vi "UI_Unlock_(02).vi"(3 "error in (no error)":errorcluster, 4 "Settings cluster in":T1={"Defaults"={"Default User"=0.0, "VISA Resource Name "=""}, "Recording and saving"={"Researcher name"="", "Name prefix"="", "Data filtering"=0, "Stop at"=0.0, "\"Stop at\" enabled"=FALSE}, "Geometry"={"Cage diameter, mm"=0, "Starting angle MIDFIELD"=0, "Starting angle BORDER"=0, "Radius, mm CENTER"=0, "Radius, mm MIDFIELD"=0, "N segments MIDFIELD"=0, "N segments BORDER"=0, "R-gap, mm"=0.0, "Bridge swap"=FALSE, "Bridge H. offset"=0.0, "Bridge V. offset"=0.0, "Twisted neck"=FALSE}, "IO parameters"={"IO general config."=0, "IO 1 configuration"=0, "IO 2 configuration"=0, "IO 3 configuration"=0, "IO 4 configuration"=0, "Activate ext. RS-232"=0, "IO inversion config."=0, "Sync capability"=1}, "Stimulus presets array"=[{"Event type"=0, "Dur., s"=0.0, "Stim., s"=0.0, "TTL out N"=1, "Set/Clear"=FALSE, "Stim. has been set"=FALSE}, {"Event type"=0, "Dur., s"=0.0, "Stim., s"=0.0, "TTL out N"=1, "Set/Clear"=FALSE, "Stim. has been set"=FALSE}, {"Event type"=0, "Dur., s"=0.0, "Stim., s"=0.0, "TTL out N"=1, "Set/Clear"=FALSE, "Stim. has been set"=FALSE}, {"Event type"=0, "Dur., s"=0.0, "Stim., s"=0.0, "TTL out N"=1, "Set/Clear"=FALSE, "Stim. has been set"=FALSE}, {"Event type"=0, "Dur., s"=0.0, "Stim., s"=0.0, "TTL out N"=1, "Set/Clear"=FALSE, "Stim. has been set"=FALSE}, {"Event type"=0, "Dur., s"=0.0, "Stim., s"=0.0, "TTL out N"=1, "Set/Clear"=FALSE, "Stim. has been set"=FALSE}, {"Event type"=0, "Dur., s"=0.0, "Stim., s"=0.0, "TTL out N"=1, "Set/Clear"=FALSE, "Stim. has been set"=FALSE}, {"Event type"=0, "Dur., s"=0.0, "Stim., s"=0.0, "TTL out N"=1, "Set/Clear"=FALSE, "Stim. has been set"=FALSE}, {"Event type"=0, "Dur., s"=0.0, "Stim., s"=0.0, "TTL out N"=1, "Set/Clear"=FALSE, "Stim. has been set"=FALSE}, {"Event type"=0, "Dur., s"=0.0, "Stim., s"=0.0, "TTL out N"=1, "Set/Clear"=FALSE, "Stim. has been set"=FALSE}, {"Event type"=0, "Dur., s"=0.0, "Stim., s"=0.0, "TTL out N"=1, "Set/Clear"=FALSE, "Stim. has been set"=FALSE}, {"Event type"=0, "Dur., s"=0.0, "Stim., s"=0.0, "TTL out N"=1, "Set/Clear"=FALSE, "Stim. has been set"=FALSE}, {"Event type"=0, "Dur., s"=0.0, "Stim., s"=0.0, "TTL out N"=1, "Set/Clear"=FALSE, "Stim. has been set"=FALSE}, {"Event type"=0, "Dur., s"=0.0, "Stim., s"=0.0, "TTL out N"=1, "Set/Clear"=FALSE, "Stim. has been set"=FALSE}], "Settings loaded OK"=FALSE} {"Stimulus presets array"."Event type" items=["Stay for N seconds"]; "Stimulus presets array"."TTL out N" items=["1"=1, "2"=2, "1+2"=3]; "Geometry"."Cage diameter, mm" scale=0.0..340.0}, 5 "All references in":T6) -> (0 "error out":errorcluster, 1 "Settings cluster out":T1={"Defaults"={"Default User"=0.0, "VISA Resource Name "=""}, "Recording and saving"={"Researcher name"="", "Name prefix"="", "Data filtering"=0, "Stop at"=0.0, "\"Stop at\" enabled"=FALSE}, "Geometry"={"Cage diameter, mm"=0, "Starting angle MIDFIELD"=0, "Starting angle BORDER"=0, "Radius, mm CENTER"=0, "Radius, mm MIDFIELD"=0, "N segments MIDFIELD"=0, "N segments BORDER"=0, "R-gap, mm"=0.0, "Bridge swap"=FALSE, "Bridge H. offset"=0.0, "Bridge V. offset"=0.0, "Twisted neck"=FALSE}, "IO parameters"={"IO general config."=0, "IO 1 configuration"=0, "IO 2 configuration"=0, "IO 3 configuration"=0, "IO 4 configuration"=0, "Activate ext. RS-232"=0, "IO inversion config."=0, "Sync capability"=1}, "Stimulus presets array"=[{"Event type"=0, "Dur., s"=0.0, "Stim., s"=0.0, "TTL out N"=1, "Set/Clear"=FALSE, "Stim. has been set"=FALSE}, {"Event type"=0, "Dur., s"=0.0, "Stim., s"=0.0, "TTL out N"=1, "Set/Clear"=FALSE, "Stim. has been set"=FALSE}, {"Event type"=0, "Dur., s"=0.0, "Stim., s"=0.0, "TTL out N"=1, "Set/Clear"=FALSE, "Stim. has been set"=FALSE}, {"Event type"=0, "Dur., s"=0.0, "Stim., s"=0.0, "TTL out N"=1, "Set/Clear"=FALSE, "Stim. has been set"=FALSE}, {"Event type"=0, "Dur., s"=0.0, "Stim., s"=0.0, "TTL out N"=1, "Set/Clear"=FALSE, "Stim. has been set"=FALSE}, {"Event type"=0, "Dur., s"=0.0, "Stim., s"=0.0, "TTL out N"=1, "Set/Clear"=FALSE, "Stim. has been set"=FALSE}, {"Event type"=0, "Dur., s"=0.0, "Stim., s"=0.0, "TTL out N"=1, "Set/Clear"=FALSE, "Stim. has been set"=FALSE}, {"Event type"=0, "Dur., s"=0.0, "Stim., s"=0.0, "TTL out N"=1, "Set/Clear"=FALSE, "Stim. has been set"=FALSE}, {"Event type"=0, "Dur., s"=0.0, "Stim., s"=0.0, "TTL out N"=1, "Set/Clear"=FALSE, "Stim. has been set"=FALSE}, {"Event type"=0, "Dur., s"=0.0, "Stim., s"=0.0, "TTL out N"=1, "Set/Clear"=FALSE, "Stim. has been set"=FALSE}, {"Event type"=0, "Dur., s"=0.0, "Stim., s"=0.0, "TTL out N"=1, "Set/Clear"=FALSE, "Stim. has been set"=FALSE}, {"Event type"=0, "Dur., s"=0.0, "Stim., s"=0.0, "TTL out N"=1, "Set/Clear"=FALSE, "Stim. has been set"=FALSE}, {"Event type"=0, "Dur., s"=0.0, "Stim., s"=0.0, "TTL out N"=1, "Set/Clear"=FALSE, "Stim. has been set"=FALSE}, {"Event type"=0, "Dur., s"=0.0, "Stim., s"=0.0, "TTL out N"=1, "Set/Clear"=FALSE, "Stim. has been set"=FALSE}], "Settings loaded OK"=FALSE} {"Stimulus presets array"."Event type" items=["Stay for N seconds"]; "Stimulus presets array"."TTL out N" items=["1"=1, "2"=2, "1+2"=3]; "Geometry"."Cage diameter, mm" scale=0.0..340.0}, 2 "All references out":T6)   [LabVIEW 2018]
uses:
  Controls/CTL_All_References.ctl
  Controls/CTL_Controls_References.ctl
  Controls/CTL_Indicators_References.ctl
  Controls/CTL_Panes_and_VIs_References.ctl
  Controls/CTL_Histogram_Properties.ctl
  <vilib>/Utility/miscctls.llb/LVRangeTypeDef.ctl
  Controls/CTL_Settings_cluster.ctl
  Controls/CTL_IO_params_cluster.ctl
  Controls/CTL_Single_stimulus_setting.ctl
  <vilib>/Utility/error.llb/Error Cluster From Error Code.vi
  <vilib>/ErrorRing/Error Ring.xnode
panel:
  in  "Histogram initialization cluster":T4={"X Scale.Range"={"Minimum"=0.0, "Maximum"=13.0, "Increment"=1.0, "Minor Increment"=1.0, "Start"=0.0}, "Caption.Text"="Zone preference (normalized)", "X Scale.Offset and Multiplier:Multiplier"=1.0, "X Scale.Offset and Multiplier:Offset"=0.0, "X Scale.Scale Fit"=2, "X Scale.Display Format:Precision"=0, "Y Scale.Mapping Mode"=0, "Zones preference empty initialized array"=[0, 0, 0, 0, 0, 0, 0, 0, 0, 0, 0, 0, 0, 0], "Plot.Fill/Point Color"=15790320}
  out "Panes references":T9
  out "Controls references params":string[][](array[string])
  out "Indicators references params":string[][](array[string])
  out "Indicators references":T8
  out "Controls references":T7
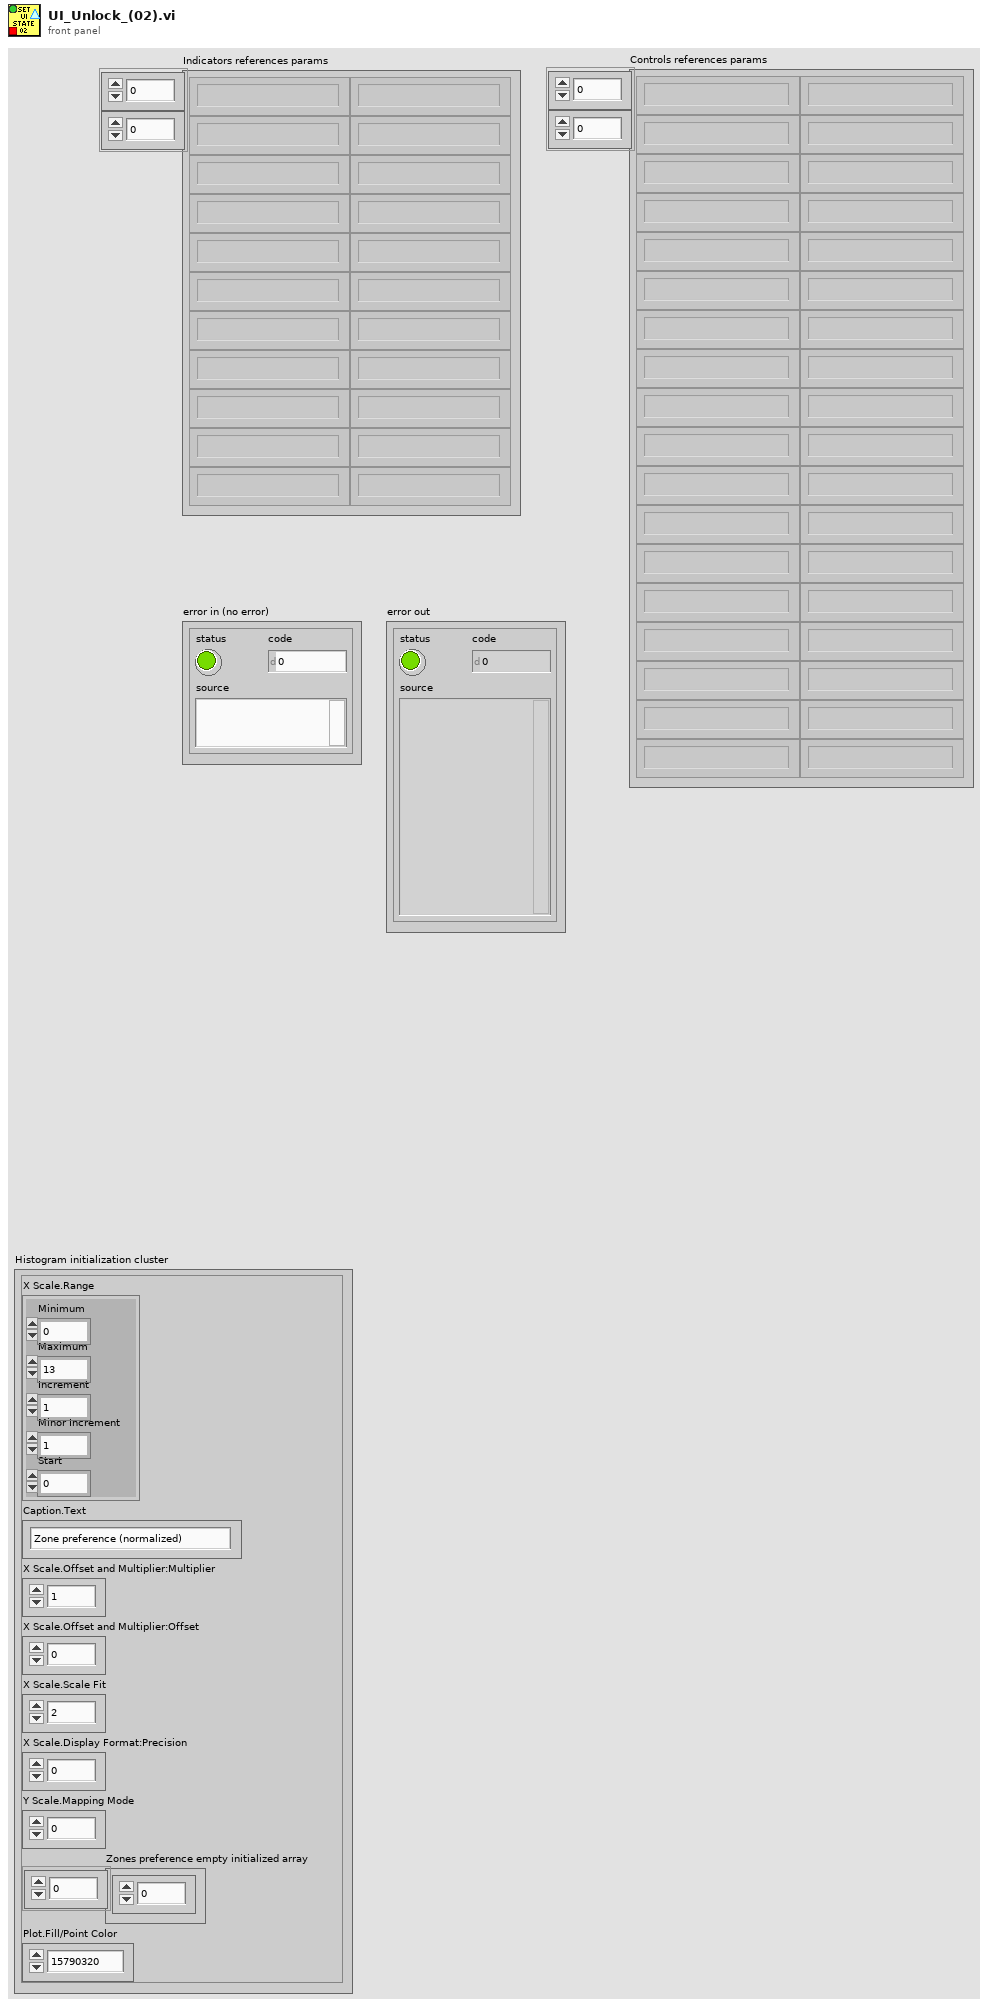
[diagram p1: front panel]
types:
  T1 = typedef "CTL_Settings_cluster.ctl" = cluster{"Defaults":cluster{"Default User":dbl, "VISA Resource Name ":string}, "Recording and saving":cluster{"Researcher name":string, "Name prefix":string, "Data filtering":u16, "Stop at":dbl, "\"Stop at\" enabled":bool}, "Geometry":cluster{"Cage diameter, mm":u16, "Starting angle MIDFIELD":i16, "Starting angle BORDER":i16, "Radius, mm CENTER":u16, "Radius, mm MIDFIELD":u16, "N segments MIDFIELD":u8, "N segments BORDER":u8, "R-gap, mm":sgl, "Bridge swap":bool, "Bridge H. offset":sgl, "Bridge V. offset":sgl, "Twisted neck":bool}, "IO parameters":T2, "Stimulus presets array":T3[], "Settings loaded OK":bool}
  T2 = typedef "CTL_IO_params_cluster.ctl" = cluster{"IO general config.":u16, "IO 1 configuration":u16, "IO 2 configuration":u16, "IO 3 configuration":u16, "IO 4 configuration":u16, "Activate ext. RS-232":u16, "IO inversion config.":u16, "Sync capability":u8}
  T3 = typedef "CTL_Single_stimulus_setting.ctl" = cluster{"Event type":u16, "Dur., s":sgl, "Stim., s":sgl, "TTL out N":u16, "Set/Clear":bool, "Stim. has been set":bool}
  T4 = typedef "CTL_Histogram_Properties.ctl" = cluster{"X Scale.Range":T5, "Caption.Text":string, "X Scale.Offset and Multiplier:Multiplier":dbl, "X Scale.Offset and Multiplier:Offset":dbl, "X Scale.Scale Fit":u8, "X Scale.Display Format:Precision":u8, "Y Scale.Mapping Mode":u8, "Zones preference empty initialized array":i32[], "Plot.Fill/Point Color":u32}
  T5 = typedef "LVRangeTypeDef.ctl" = cluster{"Minimum":dbl, "Maximum":dbl, "Increment":dbl, "Minor Increment":dbl, "Start":dbl}
  T6 = typedef "CTL_All_References.ctl" = cluster{"Controls references":T7, "Indicators references":T8, "Panes references":T9}
  T7 = typedef "CTL_Controls_References.ctl" = cluster{"Check HW connection":refnum<vi>, "Start Tracking button":refnum<vi>, "Reset zones":refnum<vi>, "Reset stimuli":refnum<vi>, "Record/Stop":refnum<vi>, "Reset barplot":refnum<vi>, "Multiplyer of chart RX":refnum<vi>, "Show zones":refnum<vi>, "Show magnets":refnum<vi>, "Show heatmap":refnum<vi>, "Show full track":refnum<vi>, "Open File":refnum<vi>, "Play/Pause":refnum<vi>, "Trace, s":refnum<vi>, "Playback speed":refnum<vi>, "Timeline":refnum<vi>, "By Zone stim. setup":refnum<vi>, "Set, Rec and Analyse Tab":refnum<vi>, "Cage radial segmentation":refnum<vi>, "Set IO config":refnum<vi>}
  T8 = typedef "CTL_Indicators_References.ctl" = cluster{"HW info":refnum<vi>, "Port":refnum<vi>, "Ready":refnum<vi>, "IO status indicator":refnum<vi>, "Current Time":refnum<vi>, "Record timestamp":refnum<vi>, "Mouse speed":refnum<vi>, "Mouse speed, mm/s":refnum<vi>, "Running, perc. of time":refnum<vi>, "Histograms":refnum<vi>}
  T9 = typedef "CTL_Panes_and_VIs_References.ctl" = cluster{"Pane":refnum<vi>, "This VI":refnum<vi>}
  T10 = cluster{"Cage diameter, mm":u16, "Starting angle MIDFIELD":i16, "Starting angle BORDER":i16, "Radius, mm CENTER":u16, "Radius, mm MIDFIELD":u16, "N segments MIDFIELD":u8, "N segments BORDER":u8, "R-gap, mm":sgl, "Bridge swap":bool, "Bridge H. offset":sgl, "Bridge V. offset":sgl, "Twisted neck":bool}
  T11 = enum8{"Enabled", "Disabled", "Disabled and Grayed Out"}
  T12 = enum32{"Page Enabled", "Page Disabled", "Page Disabled & Grayed"}
  T13 = cluster{"Radius, mm MIDFIELD":u16, "N segments MIDFIELD":u8, "Starting angle MIDFIELD":i16}
  T14 = cluster{"N segments BORDER":u8, "Starting angle BORDER":i16}
  T15 = cluster{cluster{"Radius, mm CENTER":u16}, cluster{"Radius, mm MIDFIELD":u16, "N segments MIDFIELD":u8, "Starting angle MIDFIELD":i16}, cluster{"N segments BORDER":u8, "Starting angle BORDER":i16}}
  T16 = typedef "CTL_IO_parameters_indicator.ctl" = cluster{"IO1":bool, "IO2":bool, "IO3":bool, "IO4":bool, "Z1":bool, "Z2":bool, "Z3":bool, "Z4":bool, "St1":bool, "St2":bool, "St3":bool, "St4":bool, "Syn1":bool, "Syn2":bool, "RS-232 ext. activated":bool}
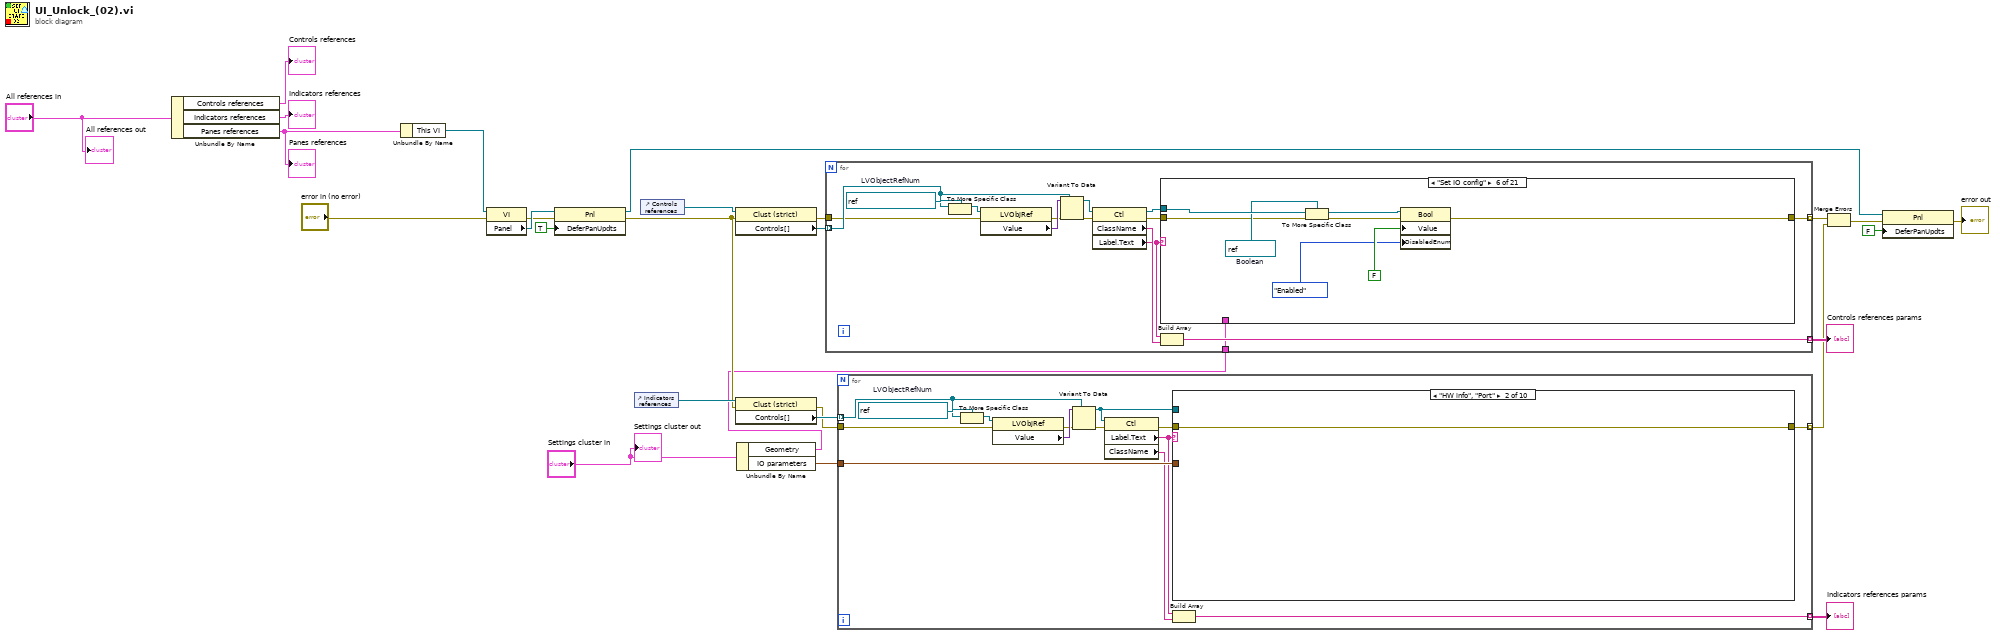
[diagram p0: block diagram]
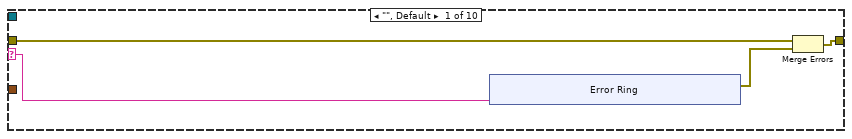
[diagram p2: hidden frame]
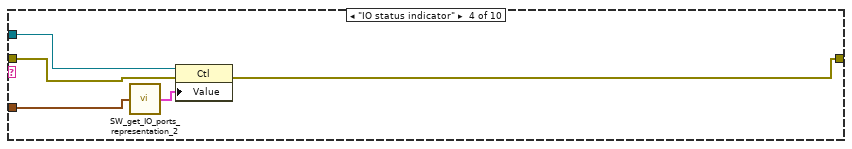
[diagram p4: hidden frame]
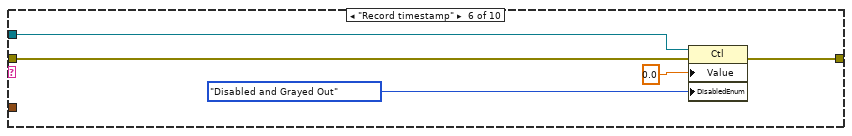
[diagram p6: hidden frame]
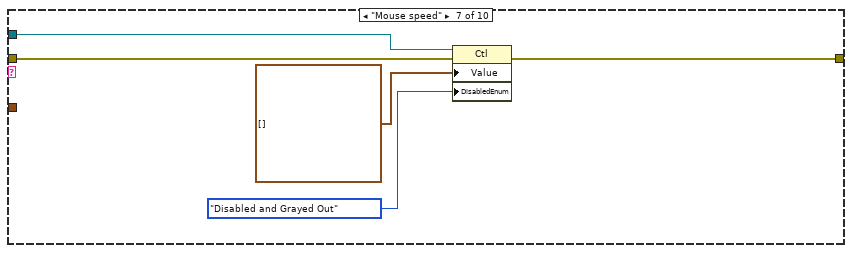
[diagram p7: hidden frame]
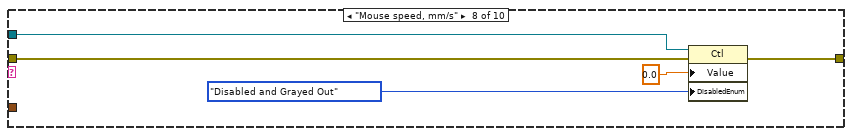
[diagram p8: hidden frame]
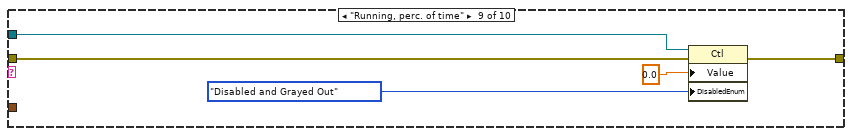
[diagram p9: hidden frame]
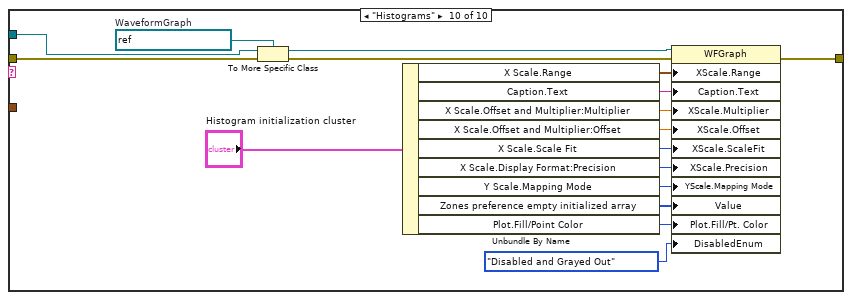
[diagram p10: hidden frame]
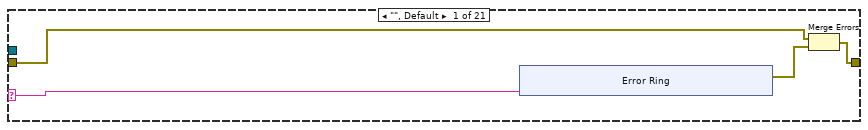
[diagram p11: hidden frame]
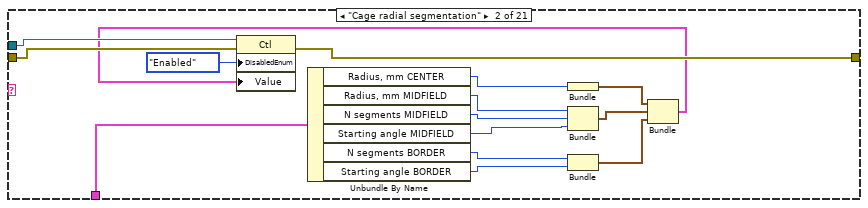
[diagram p12: hidden frame]
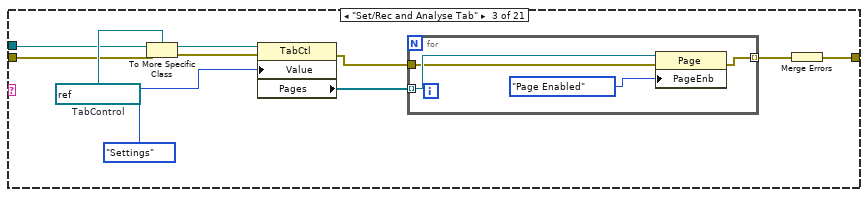
[diagram p13: hidden frame]
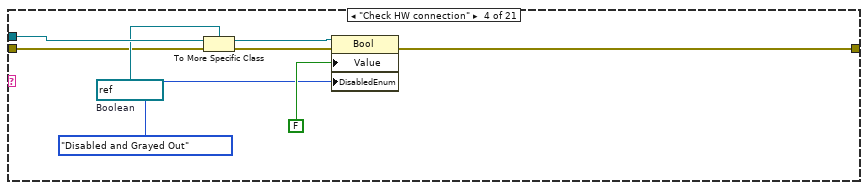
[diagram p14: hidden frame]
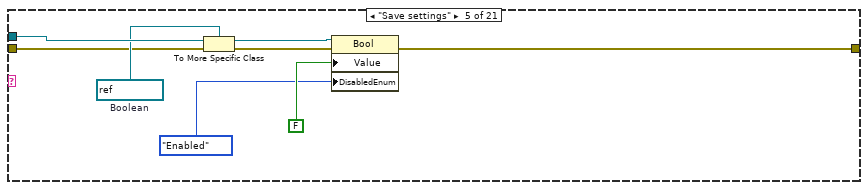
[diagram p15: hidden frame]
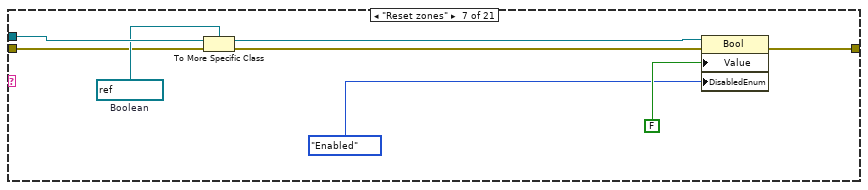
[diagram p16: hidden frame]
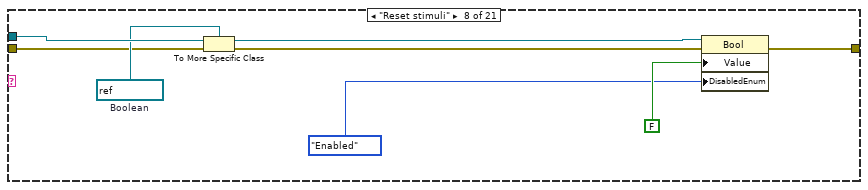
[diagram p17: hidden frame]
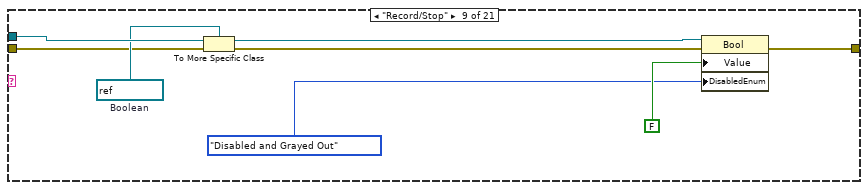
[diagram p18: hidden frame]
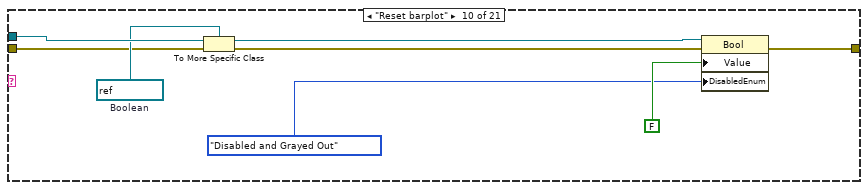
[diagram p19: hidden frame]
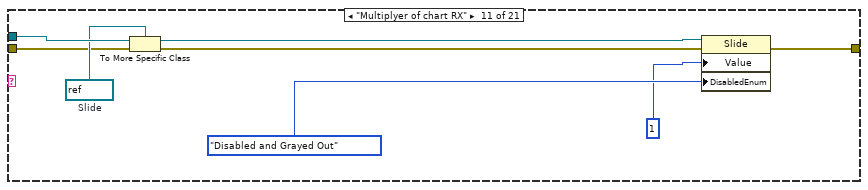
[diagram p20: hidden frame]
diagram:
  n1 = Unbundle By Name("All references in") -> ("Controls references"=→"Controls references":T7, "Indicators references"=→"Indicators references":T8, "Panes references"=w18:T9)
  "Panes references" <- w18
  n2 = Unbundle By Name(w18) -> ("This VI"=w15:refnum<vi>)
  n3 = property class="VI"(reference=w15, error in="error in (no error)") -> (error out=w7:errorcluster, "Panel"=w17:refnum<vi>)  [unwired: 1 out]
  n4 = property class="Pnl"(reference=w17, error in=w7, "DeferPanUpdts"=TRUE ("Defer Panel Updates")) -> (reference out=w8:refnum<vi>, error out=w14:errorcluster)
  n5 = control-ref of="Indicators references"() -> (w21:refnum<vi>)
  n6 = control-ref of="Controls references"() -> (w23:refnum<vi>)
  n7 = property class="Clust (strict)"(reference=w23, error in=w14) -> (error out=w13:errorcluster, "Controls[]"=w24:refnum<vi>[])  [unwired: 1 out]
  n8 = property class="Clust (strict)"(reference=w21, error in=w14) -> (error out=w12:errorcluster, "Controls[]"=w22:refnum<vi>[])  [unwired: 1 out]
  n9 = Unbundle By Name("Settings cluster in") -> ("Geometry"=w1:T10, "IO parameters"=w3:T2)
  n10 = for {
    tunnel: w24 -> [w39] mode=indexing
    tunnel: [w36] -> w19 mode=indexing
    tunnel: w13 -> [w35]
    tunnel: [w31] -> w5 mode=indexing
    tunnel: w1 -> [w28]
    w41 = refnum<vi> refnum  # LVObjectRefNum
    n11 = To More Specific Class(target class=w41, reference=w39) -> (specific class reference=w42:refnum<vi>)  [unwired: 1 in, 1 out]
    n12 = property class="LVObjRef"(reference=w42, error in=w35) -> (error out=w34:errorcluster, "Value"=w40:variant)  [unwired: 1 out]
    n13 = Variant To Data(error in=w34, type=w39, Variant=w40) -> (data=w38:refnum<vi>, error out=w33:errorcluster)
    n14 = property class="Ctl"(reference=w38, error in=w33) -> (reference out=w29:refnum<vi>, error out=w30:errorcluster, "ClassName"=w37:string, "Label.Text"=w32:string)
    n15 = case shown="\"Set IO config\"" w32 {
      selector: w32 -> [w43 _ _ _ _ _ _ _ _ _ _ _ _ _ _ _ _ _ _ _ _]
      tunnel: [w45 w66 w69 w85 w93 w101 w109 w117 w125 w133 w141 w149 w157 w165 w173 w181 w189 w197 w205 w213 w220] -> w31
      tunnel: w30 -> [w46 w67 w70 w87 w95 w103 w111 w119 w127 w135 w143 w151 w159 w167 w175 w183 w191 w199 w207 w215 w222]
      tunnel: w29 -> [_ w68 w71 w90 w98 w106 w114 w122 w130 w138 w146 w154 w162 w170 w178 w186 w194 w202 w210 w218 w225]
      tunnel: w28 -> [_ w64 _ _ _ _ _ _ _ _ _ _ _ _ _ _ _ _ _ _ _]
      frame "", Default {
        n16 = xnode "Error Ring"("parameter 0"=w43) -> ("error out"=w44:errorcluster)
        n17 = Merge Errors(w46, w44) -> (w45:errorcluster)
      }
      frame "Cage radial segmentation" {
        n18 = Unbundle By Name(w64) -> ("Radius, mm CENTER"=w63:u16, "Radius, mm MIDFIELD"=w62:u16, "N segments MIDFIELD"=w61:u8, "Starting angle MIDFIELD"=w60:i16, "N segments BORDER"=w59:u8, "Starting angle BORDER"=w58:i16)
        n19 = Bundle("Radius, mm CENTER"=w63) -> (w57:cluster{"Radius, mm CENTER":u16})  [unwired: 1 in]
        n20 = Bundle("Radius, mm MIDFIELD"=w62, "N segments MIDFIELD"=w61, "Starting angle MIDFIELD"=w60) -> (w56:T13)  [unwired: 1 in]
        n21 = Bundle("N segments BORDER"=w59, "Starting angle BORDER"=w58) -> (w55:T14)  [unwired: 1 in]
        n22 = Bundle(w57, w56, w55) -> (w54:T15)  [unwired: 1 in]
        n23 = property class="Ctl"(reference=w68, error in=w67, "DisabledEnum"=T11."Enabled" ("Disabled"), "Value"=w54) -> (error out=w66:errorcluster)  [unwired: 1 out]
      }
      frame "Set/Rec and Analyse Tab" {
        w76 = refnum<vi> refnum  # TabControl
        n24 = To More Specific Class(target class=w76, reference=w71, error in=w70) -> (specific class reference=w77:refnum<vi>, error out=w74:errorcluster)
        n25 = property class="TabCtl"(reference=w77, error in=w74, "Value"=enum32{"Settings", "Recording and Analysis"}."Settings") -> (error out=w73:errorcluster, "Pages"=w75:refnum<vi>[])  [unwired: 1 out]
        n26 = for {
          tunnel: w75 -> [w81] mode=indexing
          tunnel: w73 -> [w80]
          tunnel: [w79] -> w72 mode=indexing
          n27 = property class="Page"(reference=w81, error in=w80, "PageEnb"=T12."Page Enabled" ("Page Enabled State")) -> (error out=w79:errorcluster)  [unwired: 1 out]
        }
        n28 = Merge Errors(w72) -> (w69:errorcluster)
      }
      frame "Check HW connection" {
        w89 = refnum<vi> refnum  # Boolean
        n29 = To More Specific Class(target class=w89, reference=w90, error in=w87) -> (specific class reference=w88:refnum<vi>, error out=w86:errorcluster)
        n30 = property class="Bool"(reference=w88, error in=w86, "Value"=FALSE, "DisabledEnum"=T11."Disabled and Grayed Out" ("Disabled")) -> (error out=w85:errorcluster)  [unwired: 1 out]
      }
      frame "Save settings" {
        w97 = refnum<vi> refnum  # Boolean
        n31 = To More Specific Class(target class=w97, reference=w98, error in=w95) -> (specific class reference=w96:refnum<vi>, error out=w94:errorcluster)
        n32 = property class="Bool"(reference=w96, error in=w94, "Value"=FALSE, "DisabledEnum"=T11."Enabled" ("Disabled")) -> (error out=w93:errorcluster)  [unwired: 1 out]
      }
      frame "Set IO config" {
        w105 = refnum<vi> refnum  # Boolean
        n33 = To More Specific Class(target class=w105, reference=w106, error in=w103) -> (specific class reference=w104:refnum<vi>, error out=w102:errorcluster)
        n34 = property class="Bool"(reference=w104, error in=w102, "Value"=FALSE, "DisabledEnum"=T11."Enabled" ("Disabled")) -> (error out=w101:errorcluster)  [unwired: 1 out]
      }
      frame "Reset zones" {
        w113 = refnum<vi> refnum  # Boolean
        n35 = To More Specific Class(target class=w113, reference=w114, error in=w111) -> (specific class reference=w112:refnum<vi>, error out=w110:errorcluster)
        n36 = property class="Bool"(reference=w112, error in=w110, "Value"=FALSE, "DisabledEnum"=T11."Enabled" ("Disabled")) -> (error out=w109:errorcluster)  [unwired: 1 out]
      }
      frame "Reset stimuli" {
        w121 = refnum<vi> refnum  # Boolean
        n37 = To More Specific Class(target class=w121, reference=w122, error in=w119) -> (specific class reference=w120:refnum<vi>, error out=w118:errorcluster)
        n38 = property class="Bool"(reference=w120, error in=w118, "Value"=FALSE, "DisabledEnum"=T11."Enabled" ("Disabled")) -> (error out=w117:errorcluster)  [unwired: 1 out]
      }
      frame "Record/Stop" {
        w129 = refnum<vi> refnum  # Boolean
        n39 = To More Specific Class(target class=w129, reference=w130, error in=w127) -> (specific class reference=w128:refnum<vi>, error out=w126:errorcluster)
        n40 = property class="Bool"(reference=w128, error in=w126, "Value"=FALSE, "DisabledEnum"=T11."Disabled and Grayed Out" ("Disabled")) -> (error out=w125:errorcluster)  [unwired: 1 out]
      }
      frame "Reset barplot" {
        w137 = refnum<vi> refnum  # Boolean
        n41 = To More Specific Class(target class=w137, reference=w138, error in=w135) -> (specific class reference=w136:refnum<vi>, error out=w134:errorcluster)
        n42 = property class="Bool"(reference=w136, error in=w134, "Value"=FALSE, "DisabledEnum"=T11."Disabled and Grayed Out" ("Disabled")) -> (error out=w133:errorcluster)  [unwired: 1 out]
      }
      frame "Multiplyer of chart RX" {
        w145 = refnum<vi> refnum  # Slide
        n43 = To More Specific Class(target class=w145, reference=w146, error in=w143) -> (specific class reference=w144:refnum<vi>, error out=w142:errorcluster)
        n44 = property class="Slide"(reference=w144, error in=w142, "Value"=u8 1, "DisabledEnum"=T11."Disabled and Grayed Out" ("Disabled")) -> (error out=w141:errorcluster)  [unwired: 1 out]
      }
      frame "Show zones" {
        w153 = refnum<vi> refnum  # Boolean
        n45 = To More Specific Class(target class=w153, reference=w154, error in=w151) -> (specific class reference=w152:refnum<vi>, error out=w150:errorcluster)
        n46 = property class="Bool"(reference=w152, error in=w150, "Value"=TRUE, "DisabledEnum"=T11."Enabled" ("Disabled")) -> (error out=w149:errorcluster)  [unwired: 1 out]
      }
      frame "Show magnets" {
        w161 = refnum<vi> refnum  # Boolean
        n47 = To More Specific Class(target class=w161, reference=w162, error in=w159) -> (specific class reference=w160:refnum<vi>, error out=w158:errorcluster)
        n48 = property class="Bool"(reference=w160, error in=w158, "Value"=TRUE, "DisabledEnum"=T11."Disabled and Grayed Out" ("Disabled")) -> (error out=w157:errorcluster)  [unwired: 1 out]
      }
      frame "Show heatmap" {
        w169 = refnum<vi> refnum  # Boolean
        n49 = To More Specific Class(target class=w169, reference=w170, error in=w167) -> (specific class reference=w168:refnum<vi>, error out=w166:errorcluster)
        n50 = property class="Bool"(reference=w168, error in=w166, "Value"=FALSE, "DisabledEnum"=T11."Disabled and Grayed Out" ("Disabled")) -> (error out=w165:errorcluster)  [unwired: 1 out]
      }
      frame "Show full track" {
        w177 = refnum<vi> refnum  # Boolean
        n51 = To More Specific Class(target class=w177, reference=w178, error in=w175) -> (specific class reference=w176:refnum<vi>, error out=w174:errorcluster)
        n52 = property class="Bool"(reference=w176, error in=w174, "Value"=FALSE, "DisabledEnum"=T11."Disabled and Grayed Out" ("Disabled")) -> (error out=w173:errorcluster)  [unwired: 1 out]
      }
      frame "Open File" {
        w185 = refnum<vi> refnum  # Boolean
        n53 = To More Specific Class(target class=w185, reference=w186, error in=w183) -> (specific class reference=w184:refnum<vi>, error out=w182:errorcluster)
        n54 = property class="Bool"(reference=w184, error in=w182, "Value"=FALSE, "DisabledEnum"=T11."Enabled" ("Disabled")) -> (error out=w181:errorcluster)  [unwired: 1 out]
      }
      frame "Play/Pause" {
        w193 = refnum<vi> refnum  # Boolean
        n55 = To More Specific Class(target class=w193, reference=w194, error in=w191) -> (specific class reference=w192:refnum<vi>, error out=w190:errorcluster)
        n56 = property class="Bool"(reference=w192, error in=w190, "Value"=FALSE, "DisabledEnum"=T11."Enabled" ("Disabled")) -> (error out=w189:errorcluster)  [unwired: 1 out]
      }
      frame "Trace, s" {
        w201 = refnum<vi> refnum  # Slide
        n57 = To More Specific Class(target class=w201, reference=w202, error in=w199) -> (specific class reference=w200:refnum<vi>, error out=w198:errorcluster)
        n58 = property class="Slide"(reference=w200, error in=w198, "Value"=u8 5, "DisabledEnum"=T11."Disabled and Grayed Out" ("Disabled")) -> (error out=w197:errorcluster)  [unwired: 1 out]
      }
      frame "Playback speed" {
        w209 = refnum<vi> refnum  # Ring
        n59 = To More Specific Class(target class=w209, reference=w210, error in=w207) -> (specific class reference=w208:refnum<vi>, error out=w206:errorcluster)
        n60 = property class="Ring"(reference=w208, error in=w206, "Value"=u8 3, "DisabledEnum"=T11."Disabled and Grayed Out" ("Disabled")) -> (error out=w205:errorcluster)  [unwired: 1 out]
      }
      frame "Timeline" {
        w217 = refnum<vi> refnum  # Slide
        n61 = To More Specific Class(target class=w217, reference=w218, error in=w215) -> (specific class reference=w216:refnum<vi>, error out=w214:errorcluster)
        n62 = property class="Slide"(reference=w216, error in=w214, "Value"=u8 5, "DisabledEnum"=T11."Disabled and Grayed Out" ("Disabled")) -> (error out=w213:errorcluster)  [unwired: 1 out]
      }
      frame "By Zone stim. setup" {
        w224 = refnum<vi> refnum  # RadioButtonsControl
        n63 = To More Specific Class(target class=w224, reference=w225, error in=w222) -> (specific class reference=w223:refnum<vi>, error out=w221:errorcluster)
        n64 = property class="RadioBtnsControl"(reference=w223, error in=w221, "DisabledEnum"=T11."Enabled" ("Disabled")) -> (error out=w220:errorcluster)  [unwired: 1 out]
      }
    }
    n65 = Build Array(w32, w37) -> (w36:string[])
  }
  "Controls references params" <- w19
  n66 = for {
    tunnel: w22 -> [w236] mode=indexing
    tunnel: [w226] -> w20 mode=indexing
    tunnel: w12 -> [w234]
    tunnel: [w230] -> w11 mode=indexing
    tunnel: w3 -> [w229]
    w238 = refnum<vi> refnum  # LVObjectRefNum
    n67 = To More Specific Class(target class=w238, reference=w236) -> (specific class reference=w239:refnum<vi>)  [unwired: 1 in, 1 out]
    n68 = property class="LVObjRef"(reference=w239, error in=w234) -> (error out=w233:errorcluster, "Value"=w237:variant)  [unwired: 1 out]
    n69 = Variant To Data(error in=w233, type=w236, Variant=w237) -> (data=w235:refnum<vi>, error out=w232:errorcluster)
    n70 = property class="Ctl"(reference=w235, error in=w232) -> (error out=w231:errorcluster, "Label.Text"=w228:string, "ClassName"=w227:string)  [unwired: 1 out]
    n71 = case shown="\"HW info\", \"Port\"" w228 {
      selector: w228 -> [w240 _ _ _ _ _ _ _ _ _]
      tunnel: w235 -> [_ _ _ w254 _ w263 w268 w273 w278 w295]
      tunnel: w231 -> [w243 w251 w252 w255 w258 w262 w267 w272 w277 w281]
      tunnel: [w242 w251 w252 w257 w258 w261 w266 w271 w276 w294] -> w230
      tunnel: w229 -> [_ _ _ w256 _ _ _ _ _ _]
      frame "", Default {
        n72 = xnode "Error Ring"("parameter 0"=w240) -> ("error out"=w241:errorcluster)
        n73 = Merge Errors(w243, w241) -> (w242:errorcluster)
      }
      frame "HW info", "Port" {
      }
      frame "Ready" {
      }
      frame "IO status indicator" {
        n74 = call "SW_get_IO_ports_representation_2.vi"("Sync parameters cluster input"=w256) -> ("IO status indicator"=w253:T16)
        n75 = property class="Ctl"(reference=w254, error in=w255, "Value"=w253) -> (error out=w257:errorcluster)  [unwired: 1 out]
      }
      frame "Current Time" {
      }
      frame "Record timestamp" {
        n76 = property class="Ctl"(reference=w263, error in=w262, "Value"=0.0, "DisabledEnum"=T11."Disabled and Grayed Out" ("Disabled")) -> (error out=w261:errorcluster)  [unwired: 1 out]
      }
      frame "Mouse speed" {
        n77 = property class="Ctl"(reference=w268, error in=w267, "Value"=waveform(dbl)[] [] ("History Data"), "DisabledEnum"=T11."Disabled and Grayed Out" ("Disabled")) -> (error out=w266:errorcluster)  [unwired: 1 out]
      }
      frame "Mouse speed, mm/s" {
        n78 = property class="Ctl"(reference=w273, error in=w272, "Value"=0.0, "DisabledEnum"=T11."Disabled and Grayed Out" ("Disabled")) -> (error out=w271:errorcluster)  [unwired: 1 out]
      }
      frame "Running, perc. of time" {
        n79 = property class="Ctl"(reference=w278, error in=w277, "Value"=0.0, "DisabledEnum"=T11."Disabled and Grayed Out" ("Disabled")) -> (error out=w276:errorcluster)  [unwired: 1 out]
      }
      frame "Histograms" {
        w292 = refnum<vi> refnum  # WaveformGraph
        n80 = To More Specific Class(target class=w292, reference=w295, error in=w281) -> (specific class reference=w293:refnum<vi>, error out=w280:errorcluster)
        n81 = Unbundle By Name("Histogram initialization cluster") -> ("X Scale.Range"=w290:T5, "Caption.Text"=w289:string, "X Scale.Offset and Multiplier:Multiplier"=w288:dbl, "X Scale.Offset and Multiplier:Offset"=w287:dbl, "X Scale.Scale Fit"=w286:u8, "X Scale.Display Format:Precision"=w285:u8, "Y Scale.Mapping Mode"=w284:u8, "Zones preference empty initialized array"=w283:i32[], "Plot.Fill/Point Color"=w282:u32)
        n82 = property class="WFGraph"(reference=w293, error in=w280, "XScale.Range"=w290, "Caption.Text"=w289, "XScale.Multiplier"=w288, "XScale.Offset"=w287, "XScale.ScaleFit"=w286, "XScale.Precision"=w285, "YScale.Mapping Mode"=w284, "Value"=w283, "Plot.Fill/Pt. Color"=w282, "DisabledEnum"=T11."Disabled and Grayed Out" ("Disabled")) -> (error out=w294:errorcluster)  [unwired: 1 out]
      }
    }
    n83 = Build Array(w228, w227) -> (w226:string[])
  }
  "Indicators references params" <- w20
  n84 = Merge Errors(w5, w11) -> (w10:errorcluster)
  n85 = property class="Pnl"(reference=w8, error in=w10, "DeferPanUpdts"=FALSE ("Defer Panel Updates")) -> (error out=→"error out":errorcluster)  [unwired: 1 out]
  "All references out" <- "All references in"
  "Settings cluster out" <- "Settings cluster in"
